vi "TDK_Enable-Disable_With_Options.vi"(0 "VISA":refnum<visa-resource-name>="COM1", 1 "GEN Addr":i16=6, 2 "BAUD":u16(ring)=3 items=["1200", "2400", "4800", "9600", "19200"], 11 "error":errorcluster, 13 "Output On (T)":bool=TRUE, 14 "Settle (0 mS)":u32=1000) -> (4 "VISA out":refnum<visa-resource-name>, 15 "error out":errorcluster)   [LabVIEW 2016]
doc: "This is a simple VI to demonstrate the operation of the Lambda Genesys series DC Power Supply using the serial RS-232 or RS-485 port. This VI programs the output voltage and current, turns the output on and measures the output voltage and current.\n\nThis VI may be run as a stand-alone program if the required controls are set to the correct COM port and the power supply's address and BAUD rate. This VI may also be called as a sub-VI."
panel:
  out "code (hex)":i32 format="%.0x"
  # "Lambda Genesys \nSerial Port\n  DC Power Supplies"
  # "Getting Started:\nConfigure and Read Once"
  # "Right-Click any control\nto see it's \"Description\""
  # "WAIT"
  # "MEASURE"
  # "CONFIGURE"
  # "Right-Click to\nexplain error"
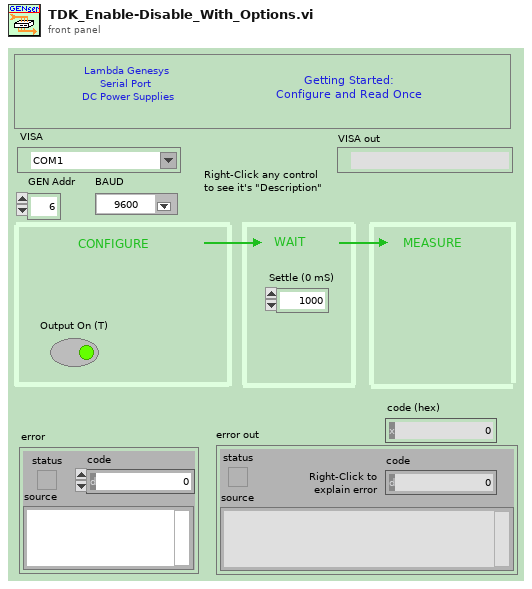
[diagram p1: front panel]
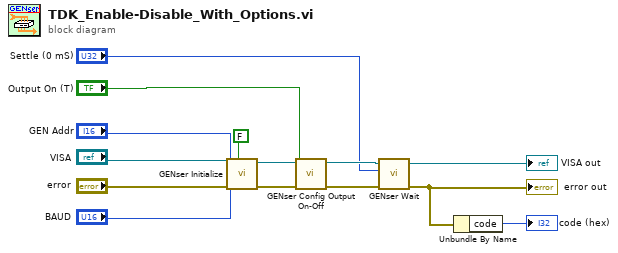
[diagram p0: block diagram]
diagram:
  n1 = call <instrlib>:"GENser Initialize.vi"("Reset (T)"=FALSE, "error in (no error)"="error", "BAUD"="BAUD", "GEN Addr"="GEN Addr", "VISA name"="VISA") -> ("error out"=w4:errorcluster, "VISA out"=w5:refnum<visa-resource-name>)  [unwired: 5 in]
  n2 = call <instrlib>:"GENser Config Output On-Off.vi"("error"=w4, "Output ON"="Output On (T)", "VISA"=w5) -> ("error out"=w11:errorcluster, "VISA out"=w12:refnum<visa-resource-name>)  [unwired: 7 in]
  n3 = call <instrlib>:"GENser Wait.vi"("error"=w11, "Delay (20 mS)"="Settle (0 mS)", "VISA"=w12) -> ("error out"=w2:errorcluster, "VISA out"=→"VISA out":refnum<visa-resource-name>)  [unwired: 7 in]
  "error out" <- w2
  n4 = Unbundle By Name(w2) -> ("code"=→"code (hex)":i32)
